vi "Wait for Daq.vi"(8 "error in (no error)":errorcluster, 11 "Recipe Process in":refnum<class "Recipe Process.lvclass">) -> (0 "error out":errorcluster, 3 "Recipe Process out":refnum<class "Recipe Process.lvclass">)   [LabVIEW 2022 SP3, in "Recipe Process.lvlib" / "Recipe Process.lvclass"]
uses:
  Recipe Process.lvclass
  Recipe Process.lvclass/Recipe Process.ctl
  XY Stage/Process Actor/Process Framework/Process State Data/Process State Data.lvclass/Process State Data.ctl
  XY Stage/Process Actor/Process Framework/Process State Data/Accessor/Read Abort.vi
  XY Stage/Process Actor/Process Framework/Process State Data/Accessor/Read Busy.vi
  IO Monitor/DAQ API/DAQ API.lvclass
  XY Stage/Process Actor/Process Framework/Process State Data/Process State Data.lvclass
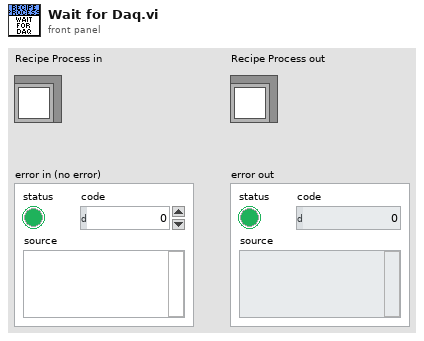
[diagram p1: front panel]
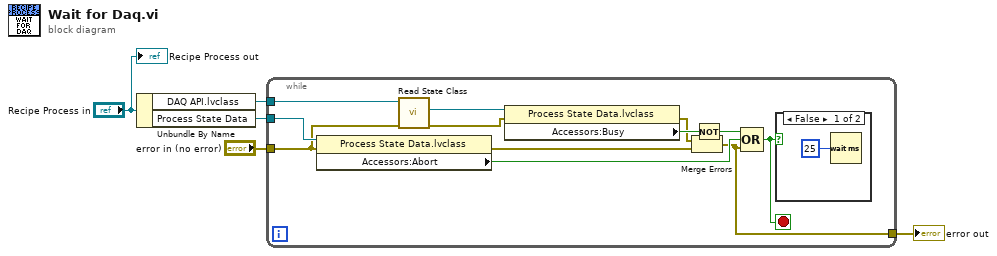
[diagram p0: block diagram]
diagram:
  n1 = Unbundle By Name("Recipe Process in") -> ("DAQ API.lvclass"=w4:refnum<class "DAQ API.lvclass">, "Process State Data"=w3:refnum<data-value>)
  n2 = while {
    tunnel: w4 -> [w17]
    tunnel: w3 -> [w15]
    tunnel: "error in (no error)" -> [w8]
    tunnel: [w9] -> w1
    stop <- w10 stop-if-true
    n3 = property class="Process State Data.lvclass"(reference=w15, error in=w8) -> (error out=w11:errorcluster, "Accessors:Abort"=w14:bool)  [unwired: 1 out]
    n4 = call-dynamic "Read State Class.vi"("error in (no error)"=w8, "Get Daq Status in"=w17) -> ("error out"=w7:errorcluster, "Process State Data"=w16:refnum<data-value>)  [unwired: 7 in, 1 out]
    n5 = property class="Process State Data.lvclass"(reference=w16, error in=w7) -> (error out=w12:errorcluster, "Accessors:Busy"=w13:bool)  [unwired: 1 out]
    n6 = Merge Errors(w12, w11) -> (w9:errorcluster)
    n7 = Not(x=w13) -> (.not. x?=w6:bool)
    n8 = Compound Arithmetic op=OR(w6, w14, w9) -> (w10:bool)
    n9 = case shown="False" w10 {
      frame False {
        n10 = Wait (ms)(milliseconds to wait=u32 25) -> ()  [unwired: 1 out]
      }
      frame True {
      }
    }
  }
  "error out" <- w1
  "Recipe Process out" <- "Recipe Process in"
